vi "Get Statistics.vi"(6 "timeout (ms)":i32=5000, 8 "error in":errorcluster, 11 "gRPC ID":T2) -> (0 "error out":errorcluster, 2 "Statistics":T1, 3 "gRPC ID out":T2)   [LabVIEW 2021, in "Template_Wrapper.lvlib"]
uses:
  Template_Wrapper.lvlib
  Template_client/Template_client.lvlib
  <vilib>/gRPC/LabVIEW gRPC Library/Shared/grpcId.ctl
  <vilib>/gRPC/LabVIEW gRPC Library/grpc-lvsupport-release.lvlib
  Template_client/RPC Messages/cif_template_GetStatisticsResponse.ctl
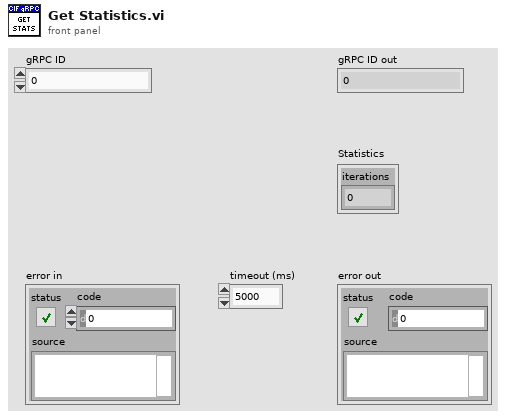
[diagram p1: front panel]
types:
  T1 = typedef "Template_client.lvlib/cif_template_GetStatisticsResponse.ctl" = cluster{"iterations":u64}
  T2 = typedef "grpc-lvsupport-release.lvlib/grpcId.ctl" = u64
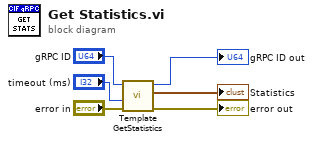
[diagram p0: block diagram]
diagram:
  n1 = call "Template GetStatistics.vi"("error in"="error in", "timeout (ms)"="timeout (ms)", "gRPC ID"="gRPC ID") -> ("error out"=→"error out":errorcluster, "Response Data"=→"Statistics":T1, "gRPC ID out"=→"gRPC ID out":T2)  [unwired: 6 in]
